vi "Pre Launch Init.vi"(11 "Display Panel V3 in":refnum<class "Display Panel V3.lvclass">) -> (0 "error out":errorcluster, 3 "Display Panel V3 out":refnum<class "Display Panel V3.lvclass">)   [LabVIEW 2014, in "Display Panel.lvlib" / "Display Panel V3.lvclass"]
doc: "(<B>Filename</B>: Actor Framework.lvlib:Actor.lvclass:Pre Launch Init.vi)\n\nDefines behavior that occurs after the Launch Actor method is invoked but before the actor's Actor Core method begins running.\n\nThe Pre Launch Init method is guaranteed to finish before the Launch Actor method returns to its caller and before the actor itself receives any messages. Any references that the Pre Launch Init method obtains are guaranteed to have the same lifetime as the actor itself. Any errors that the Pre Launch Init method returns will abort the launch.\n\nBy default, this method does nothing. A descendant class may override it to define behavior."
uses:
  Display Panel V3.lvclass
  Generic Instrument/Generic Instrument.lvclass
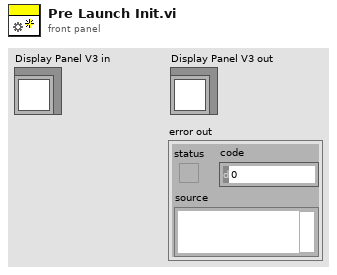
[diagram p1: front panel]
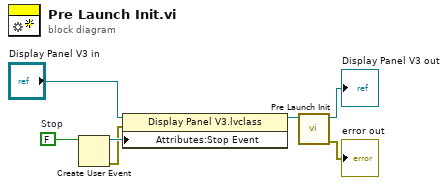
[diagram p0: block diagram]
diagram:
  w6 = FALSE  # Stop
  n1 = Create User Event(user event datatype=w6) -> (user event=w4:refnum<user-event>, error out=w3:errorcluster)  [unwired: 1 in]
  n2 = property class="Display Panel V3.lvclass"(reference="Display Panel V3 in", error in=w3, "Attributes:Stop Event"=w4) -> (reference out=w2:refnum<class "Display Panel V3.lvclass">)  [unwired: 1 out]
  n3 = call-parent "Pre Launch Init.vi"("Generic Instrument in"=w2) -> ("error out"=→"error out":errorcluster, "Generic Instrument out"=→"Display Panel V3 out":refnum<class "Display Panel V3.lvclass">)  [unwired: 9 in]
